vi "Derivative.vi"   [LabVIEW 2016, in "xy_utilities.lvlib"]
doc: "Performs numerical differentiation of the input.\n\nWire data to the data input to determine the polymorphic instance to use or manually select the instance."
uses:
  xy_utilities.lvlib
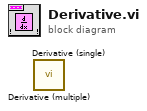
[diagram p0: block diagram]
diagram:
  n1 = call "Derivative (multiple).vi"() -> ()  [unwired: 9 in, 3 out]
  n2 = call "Derivative (single).vi"() -> ()  [unwired: 9 in, 3 out]
